vi "convert cluster to J1939 db.vi"(8 "error in":errorcluster, 10 "system db":T1, 11 "db cluster":refnum<k21>) -> (0 "error out":errorcluster)   [LabVIEW 2013, in "J1939.lvlib"]
uses:
  J1939.lvlib
  TypeDefs/J1939 db.ctl
  TypeDefs/J1939 db frame.ctl
  TypeDefs/J1939 db signal.ctl
  Internals/API Types/PGN Fields Cluster.ctl
  <vilib>/xnet/xnet.llb/XNET Database Create (Frame).vi
  <vilib>/xnet/xnet.llb/XNET Database Create (Signal).vi
  <resource>/objmgr/xnet.rc
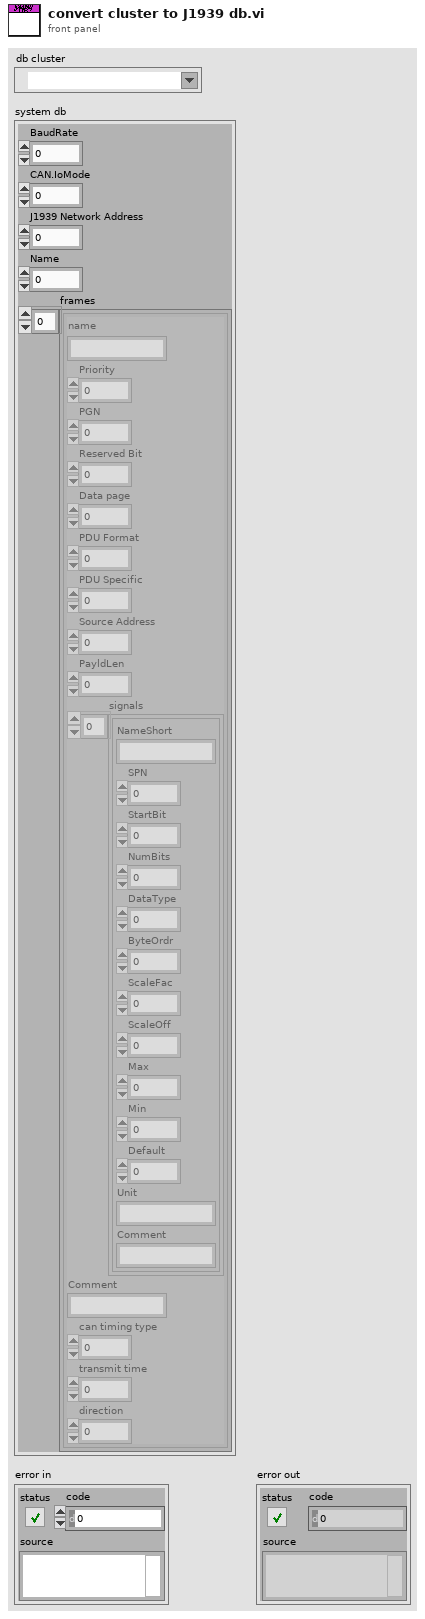
[diagram p1: front panel]
types:
  T1 = typedef "J1939.lvlib/J1939 db.ctl" = cluster{"BaudRate":u32, "CAN.IoMode":u32, "J1939 Network Address":u8, "Name":u64, "frames":T2[]}
  T2 = typedef "J1939.lvlib/J1939 db frame.ctl" = cluster{"name":string, "Priority":u8, "PGN":u32, "Reserved Bit":u8, "Data page":u8, "PDU Format":u8, "PDU Specific":u8, "Source Address":u8, "PayldLen":u32, "signals":T3[], "Comment":string, "can timing type":u32, "transmit time":dbl, "direction":u16}
  T3 = typedef "J1939.lvlib/J1939 db signal.ctl" = cluster{"NameShort":string, "SPN":i32, "StartBit":u32, "NumBits":u32, "DataType":u32, "ByteOrdr":u32, "ScaleFac":dbl, "ScaleOff":dbl, "Max":dbl, "Min":dbl, "Default":dbl, "Unit":string, "Comment":string}
  T4 = typedef "J1939.lvlib/PGN Fields Cluster.ctl" = cluster{"Reserved Bit":u8, "Data page":u8, "PDU Format":u8, "PDU Specific":u8}
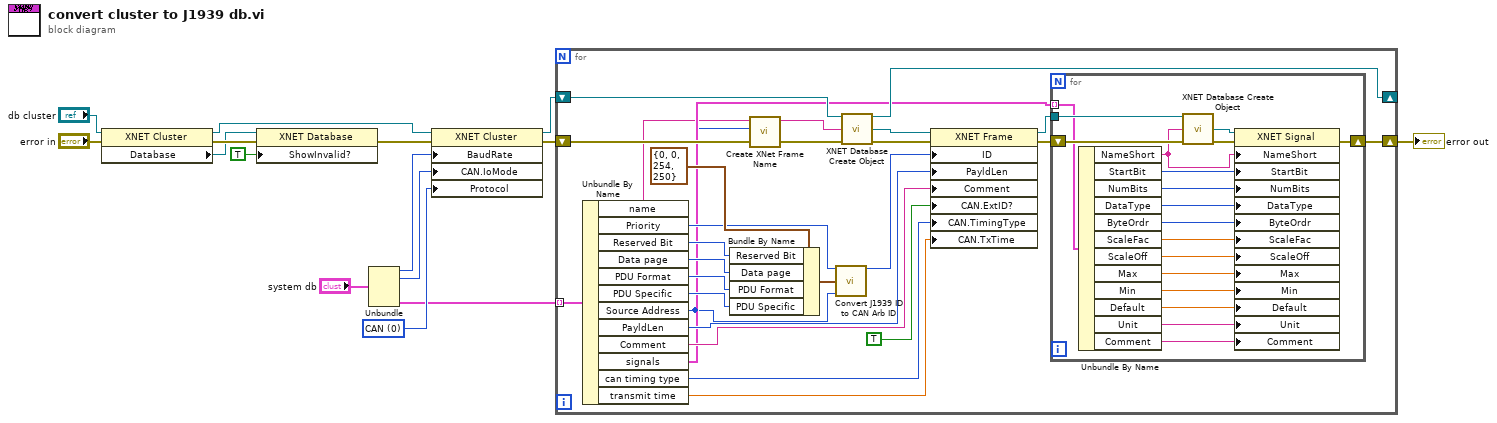
[diagram p0: block diagram]
diagram:
  w2 = u32 0 items=["CAN", "FlexRay", "LIN"] ("Protocol")
  n1 = property class="XNET Cluster"(reference="db cluster", error in="error in") -> (reference out=w9:refnum<k21>, error out=w12:errorcluster, "Database"=w11:refnum<k21>)
  n2 = property class="XNET Database"(reference=w11, error in=w12, "ShowInvalid?"=TRUE ("Show Invalid From Open?")) -> (error out=w8:errorcluster)  [unwired: 1 out]
  n3 = Unbundle("system db") -> ("BaudRate"=w7:u32, "CAN.IoMode"=w6:u32, "frames"=w1:T2[])  [unwired: 2 out]
  n4 = property class="XNET Cluster"(reference=w9, error in=w8, "BaudRate"=w7, "CAN.IoMode"=w6, "Protocol"=w2) -> (reference out=w3:refnum<k21>, error out=w5:errorcluster)
  n5 = for {
    tunnel: w1 -> [w37] mode=indexing
    shift-right: [w33] -> w4
    shift-left: w5 -> [w42]
    shift-right: [w40] -> _
    shift-left: w3 -> [w41]
    n6 = Unbundle By Name(w37) -> ("name"=w19:string, "Priority"=w24:u8, "Reserved Bit"=w27:u8, "Data page"=w28:u8, "PDU Format"=w29:u8, "PDU Specific"=w30:u8, "Source Address"=w18:u8, "PayldLen"=w36:u32, "Comment"=w35:string, "signals"=w23:T3[], "can timing type"=w16:u32, "transmit time"=w17:dbl)
    n7 = Bundle By Name(cluster=T4 {"Reserved Bit"=0, "Data page"=0, "PDU Format"=254, "PDU Specific"=250} ("PGN Fields"), "Reserved Bit"=w27, "Data page"=w28, "PDU Format"=w29, "PDU Specific"=w30) -> (w26:T4)
    n8 = call "Create XNet Frame Name.vi"("error in (no error)"=w42, "Source Address"=w18, "name"=w19) -> ("error out"=w21:errorcluster, "String"=w20:string)  [unwired: 7 in]
    n9 = call "Convert J1939 ID to CAN Arb ID.vi"("Priority"=w24, "PGN Fields"=w26, "Source Address"=w18) -> ("ID"=w25:u32)  [unwired: 11 in, 1 out]
    n10 = call-poly <vilib>:"XNET Database Create Object.vi"("cluster in"=w41, "frame name"=w20, "error in (no error)"=w21) -> ("cluster out"=w40:refnum<k21>, "frame out"=w38:refnum<k21>, "error out"=w39:errorcluster)  [unwired: 10 in]
    n11 = property class="XNET Frame"(reference=w38, error in=w39, "ID"=w25, "PayldLen"=w36, "Comment"=w35, "CAN.ExtID?"=TRUE ("CAN:Extended Identifier?"), "CAN.TimingType"=w16, "CAN.TxTime"=w17) -> (reference out=w32:refnum<k21>, error out=w34:errorcluster)
    n12 = for {
      shift-right: [w57] -> w33
      shift-left: w34 -> [w60]
      tunnel: w32 -> [w59]
      tunnel: w23 -> [w55] mode=indexing
      n13 = Unbundle By Name(w55) -> ("NameShort"=w54:string, "StartBit"=w53:u32, "NumBits"=w52:u32, "DataType"=w51:u32, "ByteOrdr"=w50:u32, "ScaleFac"=w49:dbl, "ScaleOff"=w48:dbl, "Max"=w47:dbl, "Min"=w46:dbl, "Default"=w45:dbl, "Unit"=w44:string, "Comment"=w43:string)
      n14 = call-poly <vilib>:"XNET Database Create Object.vi"("frame in"=w59, "signal name"=w54, "error in (no error)"=w60) -> ("signal out"=w56:refnum<k21>, "error out"=w58:errorcluster)  [unwired: 10 in, 1 out]
      n15 = property class="XNET Signal"(reference=w56, error in=w58, "NameShort"=w54, "StartBit"=w53, "NumBits"=w52, "DataType"=w51, "ByteOrdr"=w50, "ScaleFac"=w49, "ScaleOff"=w48, "Max"=w47, "Min"=w46, "Default"=w45, "Unit"=w44, "Comment"=w43) -> (error out=w57:errorcluster)  [unwired: 1 out]
    }
  }
  "error out" <- w4
